vi "AtDome_waitForCompletion_moveShutterDropoutDoor.vi"(8 "error in (no error)":errorcluster, 11 "waitComplete_Ctl":cluster{"cmdSeqNum":i32, "timeout":u32}) -> (0 "error out":errorcluster, 2 "function return":i32, 3 "waitComplete_Ctl out":cluster{"cmdSeqNum":i32, "timeout":u32})   [LabVIEW 2016, in "SALLV_AtDome.lvlib"]
doc: "int AtDome_shm_waitForCompletion_moveShutterDropoutDoorLV(AtDome_waitCompleteLV *waitComplete_Ctl);"
uses:
  SALLV_AtDome.lvlib
  SALLV_AtDome.so
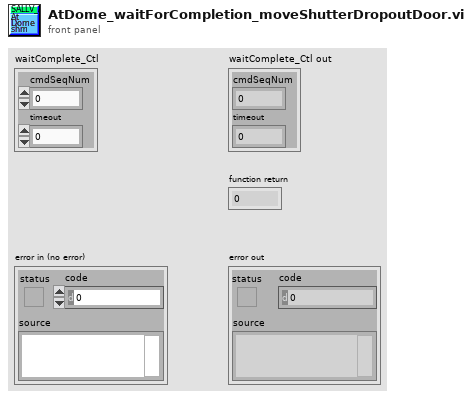
[diagram p1: front panel]
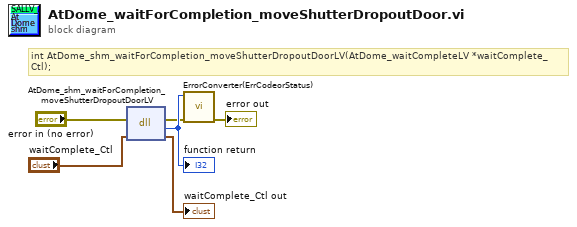
[diagram p0: block diagram]
diagram:
  # "int AtDome_shm_waitForCompletion_moveShutterDropoutDoorLV(AtDome_waitCompleteLV *waitComplete_Ctl);"
  n1 = dll-call lib="home/andres/Desktop/SAL_AtDome/SALLV_AtDome.*" fn="AtDome_shm_waitForCompletion_moveShutterDropoutDoorLV"(error in="error in (no error)", "waitComplete_Ctl"="waitComplete_Ctl") -> (error out=w2:errorcluster, w6:i32, "waitComplete_Ctl"=→"waitComplete_Ctl out":cluster{"cmdSeqNum":i32, "timeout":u32})  [unwired: 2 in, 1 out]
  "function return" <- w6
  n2 = call "ErrorConverter(ErrCodeorStatus).vi"("error in (no error)"=w2, "error code"=w6) -> ("error out"=→"error out":errorcluster)  [unwired: 9 in]
